vi "Epoxy_Main.vi"() -> ()   [LabVIEW 2020]
doc: "This template is for the Queued Message Handler design pattern.\n\nThe Event Handling Loop generates messages based on user interface actions.\n\nThe Message Handling Loop processes messages generated by the Event Handling Loop, or by other messages. The messages are string values, so new messages can be added easily to the Message Cases case structure in the Message Handling Loop. Each message cluster can also provide an optional value for Message Data, which is a variant that can be converted to whatever message-specific data is required."
uses:
  controls/UI Data.ctl
  DAQLoop_Typedef.ctl
  controls/Data Loop Enum.ctl
  controls/DAQ FGV.ctl
  <vilib>/Utility/error.llb/DialogType.ctl
  controls/Valve Timer FGV.ctl
  controls/SaveTimer.ctl
  Global Loop Stop.vi
  Global Zero or Not Ctrl.vi
  Global Zero Constants.vi
  support/Message Queue/Enqueue Message (Single).vi
  <vilib>/Utility/error.llb/Error Cluster From Error Code.vi
  <vilib>/ErrorRing/Error Ring.xnode
  support/Message Queue/Message Queue.lvlib
  support/User Event - Stop/User Event - Stop.lvlib
  <instrlib>/Agilent 34970/Agilent 34970.lvlib
panel:
  out "T 7":dbl format="%.2f"
  out "T 6":dbl format="%.2f"
  out "T 5":dbl format="%.2f"
  out "T 4":dbl format="%.2f"
  out "T 3":dbl format="%.2f"
  out "T 2":dbl format="%.2f"
  out "T 1":dbl format="%.2f"
  out "Time":string
  out "DAQ":bool
  out "State Execution (ms)":u32=250 format="%.0p"
  out "Messages":string
  out "Lap":dbl format="%<%H:%M:%S>t"
  in  "Interval":dbl=5.0 min=0.0 max=5.0 step=1.0 format="%.2f s"
  in  "FileName":string="Epoxy_"
  in  "Save Command":bool
  in  "Tab Control":enum32{"GRAPH", "OTHER"}(tab)
  in  "Run Interval":dbl=1.0 format="%.1f min"
  in  "Run Auto":bool
  in  "Run B":bool
  in  "Run A":bool
  in  "Axis Update":bool
  out "Waveform Chart Out":dynamicdata(graph)
  in  "Minutes X-axis":dbl format="%#_g min"
  out "Count Down":dbl format="%<%H:%M:%S>t"
  in  "milliseconds DAQ Loop":u32=1000
  in  "Scan List":string="101,102,103,104,105,106,107"
  in  "Transducer Type":T1(ring)
  in  "Thermocouple Type":T2(ring)=enum."T"
  in  "VISA resource name":refnum<visa-resource-name>="COM6"
  out "M1":dbl[](array[numeric])
  in  "Serial Port Configuration":T3={"Timeout Value (10000)"=10000, "Baud Rate (57600)"=enum."9600", "Flow Control (1:XON/XOFF)"=enum."XON / XOFF"}
  in  "Reset (T: Reset)":bool=TRUE
  in  "Save File Headers":string[](array[string])=["T1", "T2", "T3", "T4", "T5", "T6", "T7"]
  in  "Exit":bool
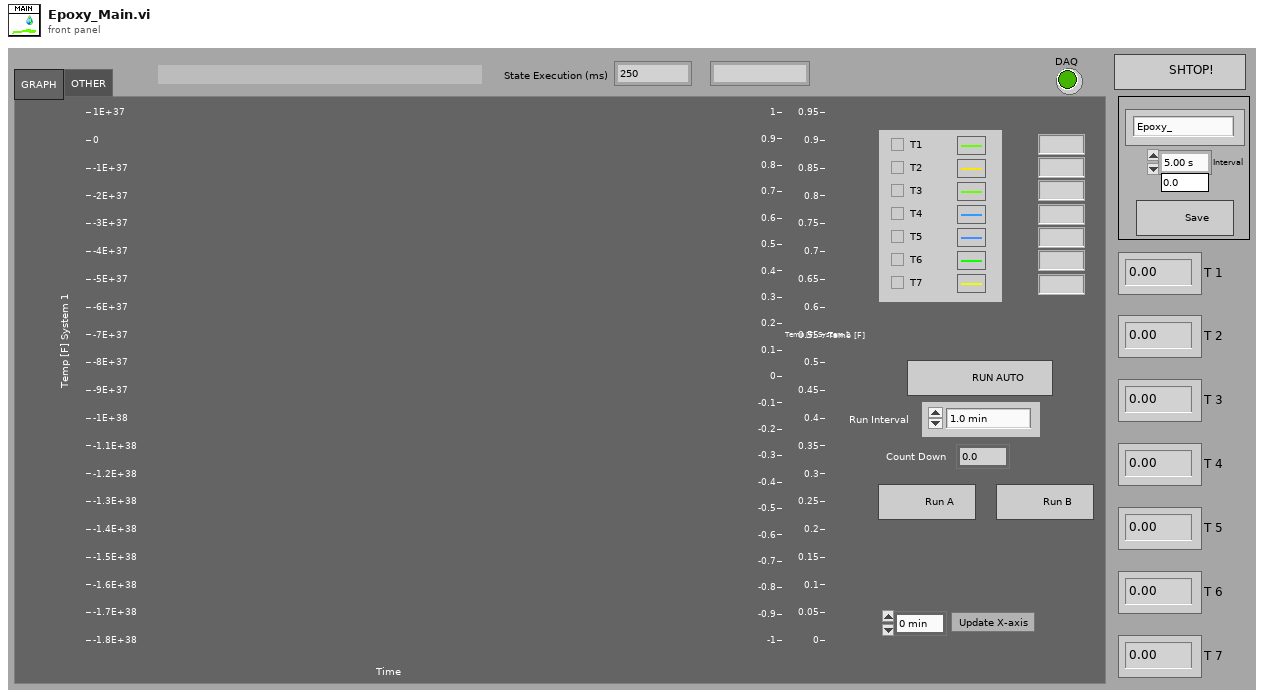
[diagram p1: front panel]
types:
  T1 = enum16{"Thermocouple", "Thermistor", "RTD", "4-Wire RTD", "Default (Last)"}
  T2 = enum16{"B", "E", "J", "K", "N", "R", "S", "T", "Default (Last)"}
  T3 = cluster{"Timeout Value (10000)":u32, "Baud Rate (57600)":enum16{"1200", "2400", "4800", "9600", "19200", "38400", "57600", "115200"}, "Flow Control (1:XON/XOFF)":enum16{"None", "XON / XOFF", "RTS / CTS", "DTR / DSR"}}
  T4 = typedef "Data Loop Enum.ctl" = enum16{"Initialize", "Run", "Exit"}
  T5 = typedef "DAQLoop_Typedef.ctl" = cluster{"XL time":dbl, "Temps":cluster{"TC_1":dbl, "TC_ 2":dbl, "TC_ 3":dbl, "TC_ 4":dbl, "TC_ 5":dbl, "TC_ 6":dbl, "TC_ 7":dbl}}
  T6 = typedef "UI Data.ctl" = cluster{"VISA ref":refnum<visa-resource-name>, "SavePath":path, "tdms file out":refnum<k34>}
  T7 = typedef "Message Queue.lvlib/All Message Queues.ctl" = cluster{"UI":refnum<queue>}
  T8 = typedef "DAQ FGV.ctl" = enum16{"Read", "Pass"}
  T9 = typedef "DialogType.ctl" = u16
  T10 = typedef "Valve Timer FGV.ctl" = enum16{"Run", "Check", "Stop"}
  T11 = typedef "SaveTimer.ctl" = enum16{"Start Save", "StartInterval", "UpdateInterval", "Check"}
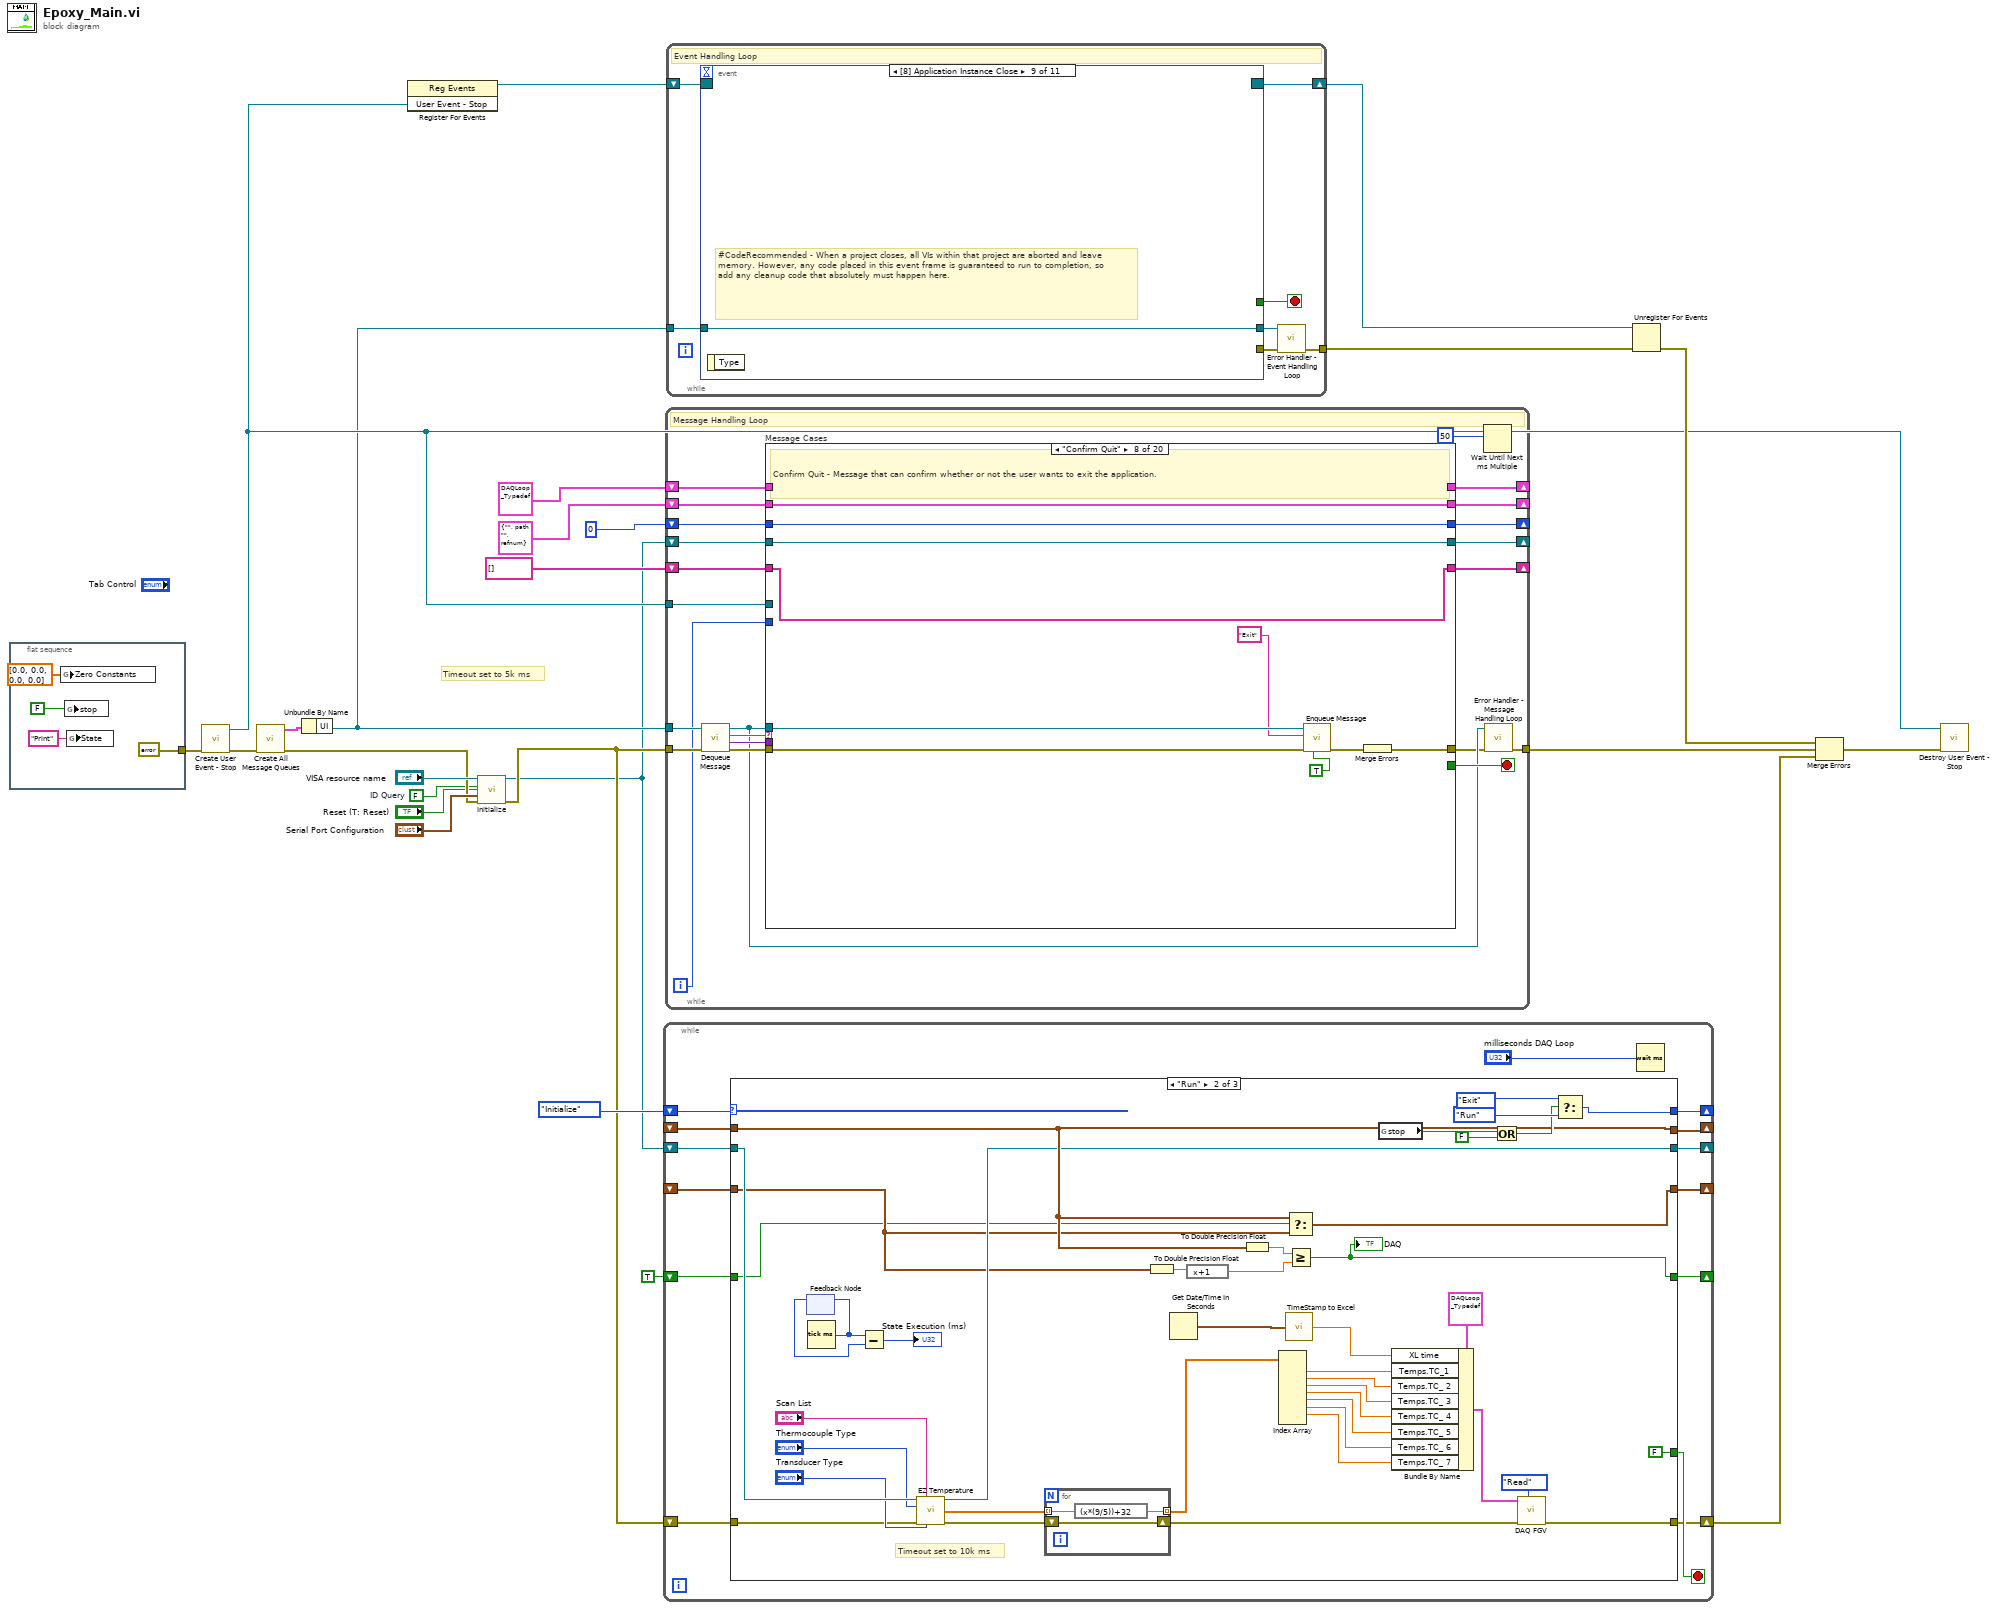
[diagram p0: block diagram]
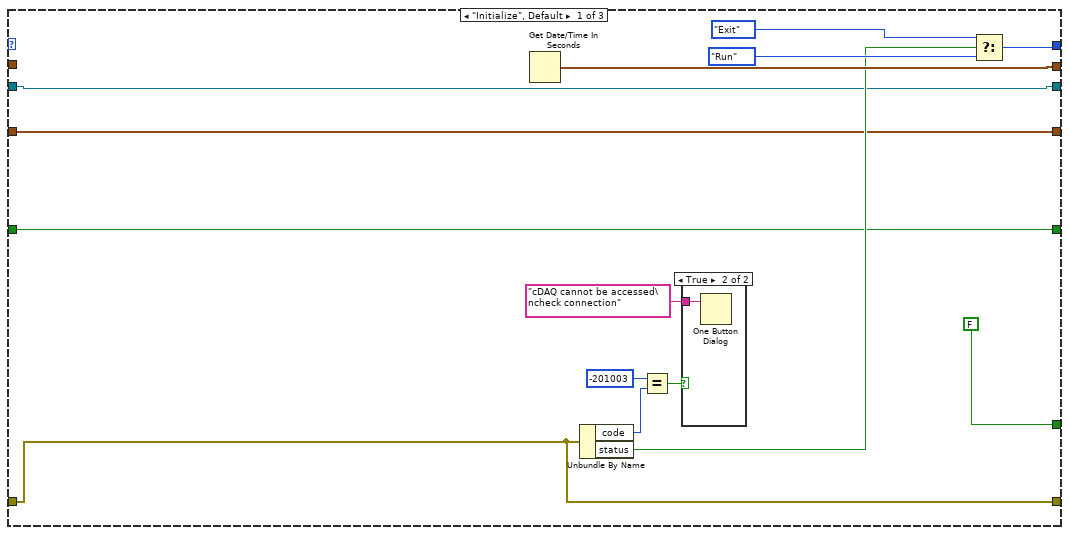
[diagram p2: hidden frame]
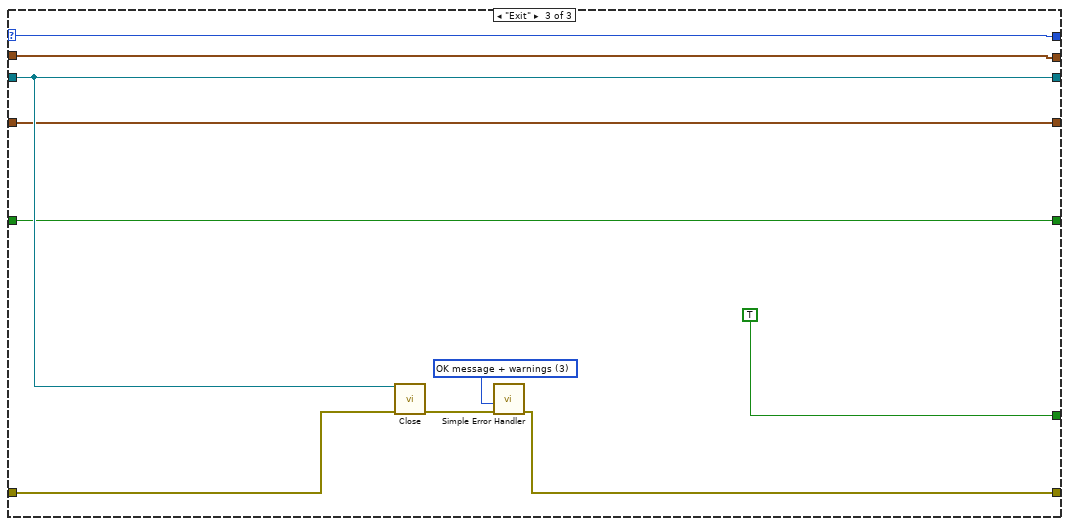
[diagram p4: hidden frame]
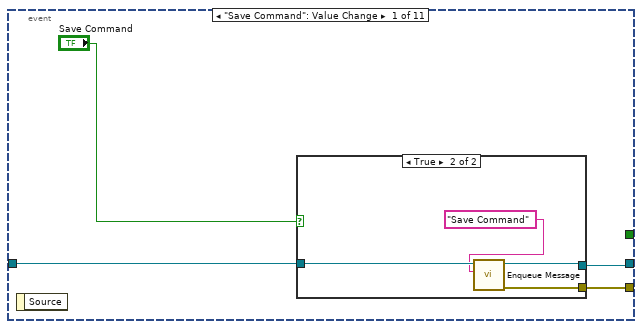
[diagram p5: hidden frame]
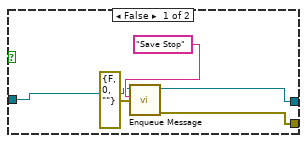
[diagram p6: hidden frame]
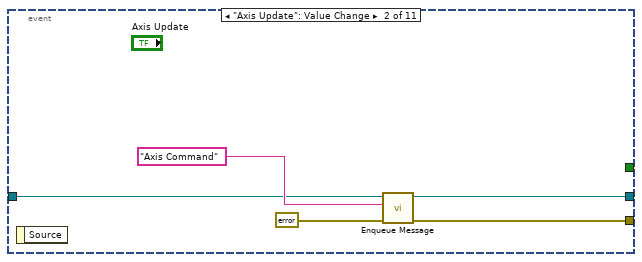
[diagram p7: hidden frame]
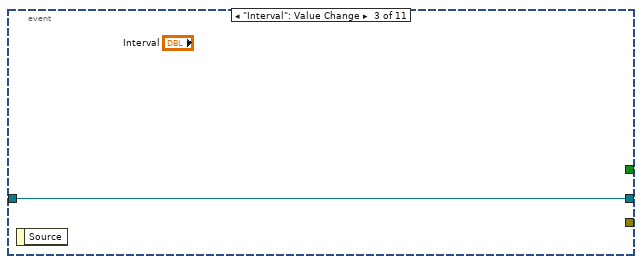
[diagram p8: hidden frame]
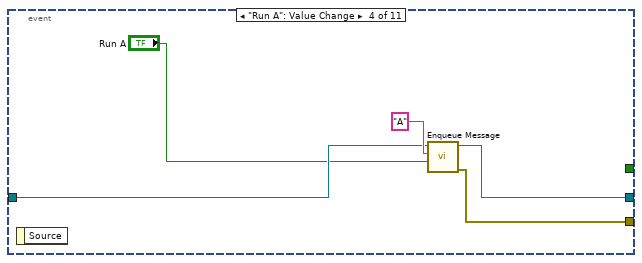
[diagram p9: hidden frame]
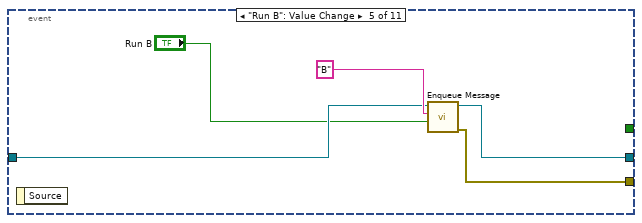
[diagram p10: hidden frame]
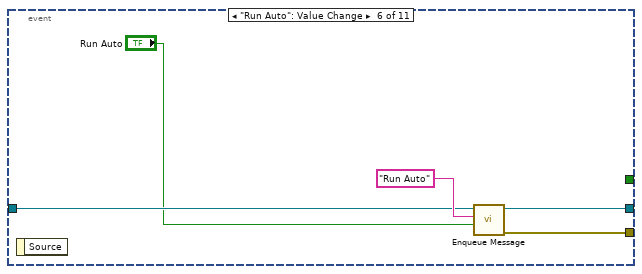
[diagram p11: hidden frame]
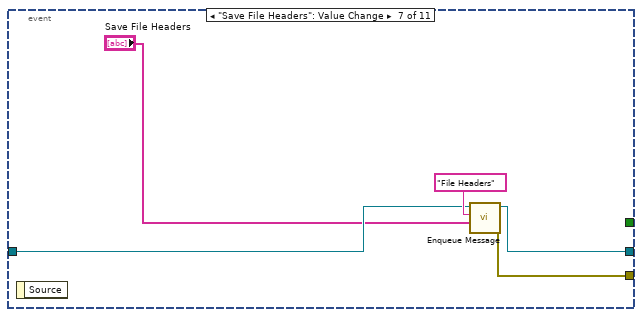
[diagram p12: hidden frame]
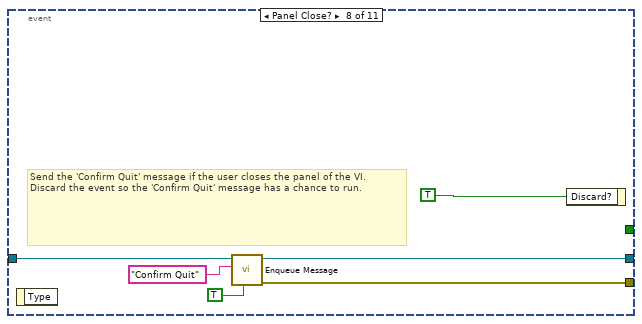
[diagram p13: hidden frame]
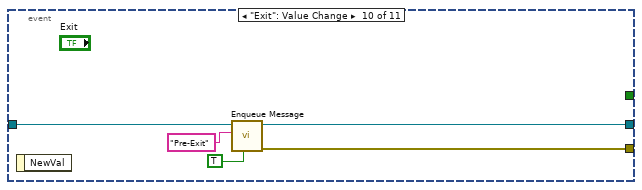
[diagram p14: hidden frame]
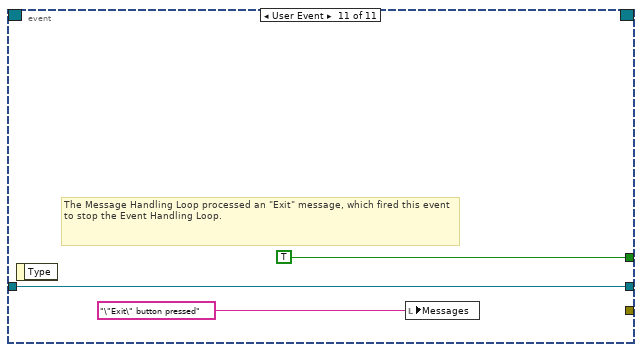
[diagram p15: hidden frame]
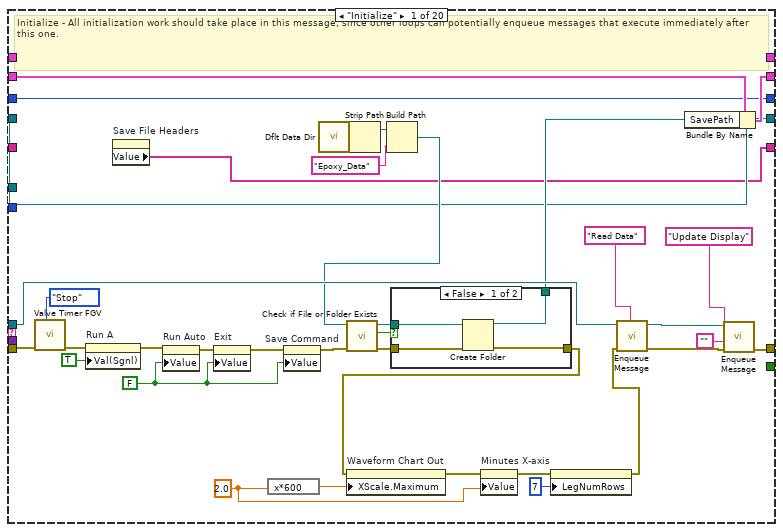
[diagram p16: hidden frame]
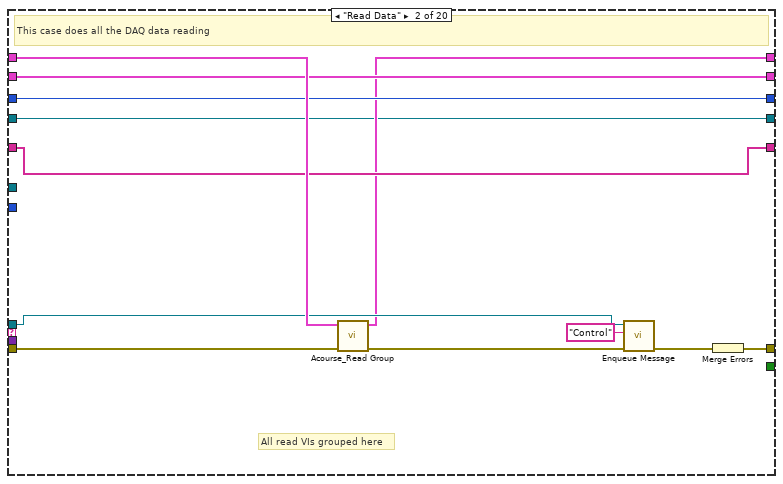
[diagram p18: hidden frame]
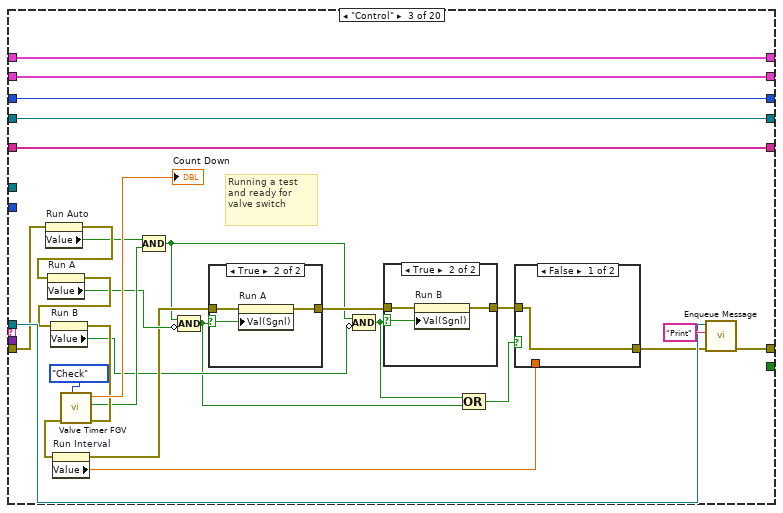
[diagram p19: hidden frame]
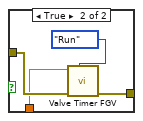
[diagram p20: hidden frame]
diagram:
  w2 = FALSE  # ID Query
  # "Timeout set to 5k ms"
  n1 = flat-sequence {
    tunnel: [errorcluster {"status"=FALSE, "code"=0, "source"=""} ("error out")] -> w16
    frame #0 {
      n2 = global write "Global Zero Constants.vi" "Zero Constants"(dbl[] [0.0, 0.0, 0.0, 0.0] ("Zero Constants")) -> ()
      n3 = global write "Global Loop Stop.vi" "stop"(FALSE ("stop")) -> ()
      n4 = global write "Global Zero or Not Ctrl.vi" "State"("Print" ("State")) -> ()
    }
  }
  n5 = call "Create User Event - Stop.vi"("error in (no error)"=w16) -> ("error out"=w23:errorcluster, "User Event - Stop"=w17:refnum<user-event>)  [unwired: 9 in]
  n6 = call "Create All Message Queues.vi"("error in (no error)"=w23) -> ("error out"=w7:errorcluster, "Message Queues out"=w25:T7)  [unwired: 9 in]
  n7 = Unbundle By Name(w25) -> ("UI"=w15:refnum<queue>)
  n8 = register-events(w17) -> (reference out=w18:refnum<event-registration>)  [unwired: 2 in, 1 out]
  n9 = call <instrlib>:"Initialize.vi"("VISA Resource Name"="VISA resource name", "ID Query (T: Check)"=w2, "Reset (T: Reset)"="Reset (T: Reset)", "Serial Port Configuration"="Serial Port Configuration", "error in (no error)"=w7) -> ("VISA Resource Name Out"=w5:refnum<visa-resource-name>, "error out"=w6:errorcluster)  [unwired: 9 in]
  n10 = while {
    shift-right: [w42] -> _
    shift-left: Data_Loop_Enum."Initialize" ("Enum") -> [w43]
    shift-right: [w34] -> _
    shift-left: w5 -> [w37]
    shift-right: [w36] -> w13
    shift-left: w6 -> [w35]
    shift-right: [w41] -> _
    shift-left: _ -> [w40]
    shift-right: [w32] -> _
    shift-left: _ -> [w33]
    shift-right: [w30] -> _
    shift-left: TRUE -> [w31]
    stop <- w39 stop-if-true
    n11 = case shown="\"Run\"" w43 {
      selector: w43 -> [_ _ w112]
      tunnel: [w47 w91 w107] -> w36
      tunnel: [w46 w77 w106] -> w34
      tunnel: [w55 w92 w112] -> w42
      tunnel: [w54 w84 w111] -> w41
      tunnel: w40 -> [_ w84 w111]
      tunnel: [FALSE FALSE TRUE] -> w39
      tunnel: w37 -> [w46 w80 w106]
      tunnel: w35 -> [w47 w67 w105]
      tunnel: w33 -> [w44 w62 w103]
      tunnel: [w44 w61 w103] -> w32
      tunnel: w31 -> [w45 w60 w104]
      tunnel: [w45 w59 w104] -> w30
      frame "Initialize", Default {
        n12 = Get Date/Time In Seconds() -> (seconds since 1Jan1904=w54:timestamp)
        n13 = Unbundle By Name(w47) -> ("code"=w49:i32, "status"=w48:bool)
        n14 = Equal?(x=-201003, y=w49) -> (x = y?=w51:bool)
        n15 = case shown="True" w51 {
          tunnel: "cDAQ cannot be accessed\ncheck connection" ("message") -> [_ w58]
          frame False {
          }
          frame True {
            n16 = One Button Dialog(message=w58) -> ()  [unwired: 1 in, 1 out]
          }
        }
        n17 = Select(t=Data_Loop_Enum."Exit", s=w48, f=Data_Loop_Enum."Run") -> (s? t:f=w55:T4)
      }
      frame "Run" {
        # "Timeout set to 10k ms"
        n18 = feedback #1() -> (w96:u32)  [unwired: 1 in]
        n19 = Tick Count (ms)() -> (millisecond timer value=w95:u32)
        n20 = feedback-in #1(w95) -> ()
        n21 = Subtract(x=w95, y=w96) -> (x-y=→"State Execution (ms)":u32)
        n22 = call <instrlib>:"EZ Temperature.vi"("VISA Resource Name"=w80, "Scan List (empty)"="Scan List", "Thermocouple Type (8:Def-Last)"="Thermocouple Type", "error in (no error)"=w67, "Transducer Type (4:Def-Last)"="Transducer Type") -> ("VISA Resource Name Out"=w77:refnum<visa-resource-name>, "Output Array"=w64:dbl[], "error out"=w66:errorcluster)  [unwired: 8 in]
        n23 = for {
          shift-right: [w102] -> w65
          shift-left: w66 -> [w102]
          tunnel: w64 -> [w101] mode=indexing
          tunnel: [w100] -> w63 mode=indexing
          n24 = expression code="(x*(9/5))+32"(w101) -> (w100:dbl)
        }
        n25 = To Double Precision Float(number=w62) -> (double precision float=w99:dbl)
        n26 = Get Date/Time In Seconds() -> (seconds since 1Jan1904=w83:timestamp)
        n27 = expression code="x+1"(w99) -> (w97:dbl)
        n28 = To Double Precision Float(number=w84) -> (double precision float=w98:dbl)
        n29 = Index Array(array=w63) -> (element #1=w75:dbl, element #2=w74:dbl, element #3=w73:dbl, element #4=w72:dbl, element #5=w71:dbl, element #6=w70:dbl, element #7=w69:dbl)  [unwired: 8 in, 1 out]
        n30 = call "TimeStamp to Excel.vi"("Time Stamp"=w83) -> ("XL Time"=w68:dbl)
        n31 = Select(t=w84, s=w60, f=w62) -> (s? t:f=w61:timestamp)
        n32 = Greater Or Equal?(x=w98, y=w97) -> (x >= y?=w59:bool)
        "DAQ" <- w59
        n33 = global read "Global Loop Stop.vi" "stop"() -> (w87:bool)
        n34 = Bundle By Name(cluster=T5 {"XL time"=0.0, "Temps"={"TC_1"=0.0, "TC_ 2"=0.0, "TC_ 3"=0.0, "TC_ 4"=0.0, "TC_ 5"=0.0, "TC_ 6"=0.0, "TC_ 7"=0.0}} ("Cluster"), "XL time"=w68, "Temps.TC_1"=w75, "Temps.TC_ 2"=w74, "Temps.TC_ 3"=w73, "Temps.TC_ 4"=w72, "Temps.TC_ 5"=w71, "Temps.TC_ 6"=w70, "Temps.TC_ 7"=w69) -> (w85:T5)
        n35 = Or(x=w87, y=FALSE) -> (x .or. y?=w89:bool)
        n36 = call "DAQ FGV.vi"("Enum"=DAQ_FGV."Read", "error in (no error)"=w65, "Cluster"=w85) -> ("error out"=w91:errorcluster)  [unwired: 7 in, 1 out]
        n37 = Select(t=Data_Loop_Enum."Exit", s=w89, f=Data_Loop_Enum."Run") -> (s? t:f=w92:T4)
      }
      frame "Exit" {
        w109 = T9 3 items=["no dialog", "OK message", "continue or stop message", "OK message + warnings", "continue/stop + warnings"] ("type of dialog (OK msg:1)")
        n38 = call <instrlib>:"Close.vi"("VISA Resource Name"=w106, "error in (no error)"=w105) -> ("error out"=w108:errorcluster)  [unwired: 13 in]
        n39 = call <vilib>:"Simple Error Handler.vi"("type of dialog (OK msg:1)"=w109, "error in (no error)"=w108) -> ("error out"=w107:errorcluster)  [unwired: 3 in, 4 out]
      }
    }
    n40 = Wait (ms)(milliseconds to wait="milliseconds DAQ Loop") -> ()  [unwired: 1 out]
  }
  n41 = while {
    tunnel: w15 -> [w126]
    shift-right: [w133] -> _
    shift-left: T6 {"VISA ref"="", "SavePath"=path "", "tdms file out"=refnum} ("Data Cluster") -> [w134]
    tunnel: w17 -> [w131]
    tunnel: w6 -> [w130]
    tunnel: [w124] -> w24
    shift-right: [w121] -> _
    shift-left: T5 {"XL time"=0.0, "Temps"={"TC_1"=0.0, "TC_ 2"=0.0, "TC_ 3"=0.0, "TC_ 4"=0.0, "TC_ 5"=0.0, "TC_ 6"=0.0, "TC_ 7"=0.0}} ("Cluster") -> [w122]
    shift-right: [w117] -> _
    shift-left: 0 -> [w118]
    shift-right: [w115] -> _
    shift-left: string[] [] ("appended array") -> [w116]
    shift-right: [w113] -> _
    shift-left: w5 -> [w114]
    i -> [w119]
    stop <- w132 stop-if-true
    # "Message Handling Loop"
    n42 = call "Dequeue Message.vi"("error in (no error)"=w130, "Message Queue"=w126) -> ("error out"=w129:errorcluster, "Message Data"=w127:variant, "Message"=w128:string, "dup Message Queue"=w125:refnum<queue>)  [unwired: 6 in]
    n43 = case "Message Cases" shown="\"Confirm Quit\"" w128 {
      selector: w128 -> [_ _ _ _ _ _ _ _ _ _ _ _ _ _ _ _ _ _ _ w489]
      tunnel: w125 -> [w169 w184 w208 w257 w279 _ _ w319 _ _ _ _ _ _ w412 w421 _ w451 w484 _]
      tunnel: w129 -> [w137 w188 w207 w253 w274 w299 w312 w323 w330 w339 w356 w372 w383 w393 w411 w422 w440 w449 w479 _]
      tunnel: [w165 w189 w211 w258 w280 w300 w306 w321 w328 w343 w360 w376 w386 w397 w413 w423 w434 w452 w482 w490] -> w123
      tunnel: w134 -> [w163 w183 w217 w259 w289 w301 w311 w322 w329 w344 w361 w377 w387 w398 w403 w430 w439 w450 w473 w491]
      tunnel: [w162 w183 w217 w259 w289 w301 w311 w322 w329 w344 w361 w377 w387 w398 w402 w430 w439 w450 w473 w491] -> w133
      tunnel: [_ _ _ _ _ _ _ _ _ _ _ _ _ _ _ _ _ _ TRUE _] -> w132
      tunnel: w127 -> [_ _ _ _ _ w298 w310 _ _ _ w355 w371 w382 _ _ _ _ _ w476 _]
      tunnel: w131 -> [_ _ _ _ _ _ _ _ _ _ _ _ _ _ _ _ _ _ w481 _]
      tunnel: w122 -> [w171 w187 w216 w250 w290 w295 w305 w316 w327 w342 w359 w375 w385 w396 w417 w429 w441 w454 w474 w488]
      tunnel: [w171 w180 w216 w250 w290 w295 w305 w316 w327 w342 w359 w375 w385 w396 w417 w429 w441 w454 w474 w488] -> w121
      tunnel: w119 -> [_ _ _ _ _ _ _ _ _ _ _ _ _ _ _ w427 _ _ _ _]
      tunnel: w118 -> [w143 w182 w215 w255 w277 w293 w304 w315 w326 w341 w358 w374 w384 w395 w401 _ w433 w448 w472 w487]
      tunnel: [w143 w182 w215 w255 w277 w293 w304 w315 w326 w341 w358 w374 w384 w395 w401 w425 w433 w448 w472 w487] -> w117
      tunnel: w116 -> [_ w181 w214 w237 w276 w292 w303 w314 w325 w340 w357 w373 _ w390 w400 w419 w432 w447 w471 w486]
      tunnel: [w135 w181 w214 w237 w276 w292 w303 w314 w325 w340 w357 w373 w378 w390 w400 w419 w432 w447 w471 w486] -> w115
      tunnel: w114 -> [w144 w179 w213 w231 w275 w291 w302 w313 w324 w333 w348 w369 w381 w389 w399 w418 w431 w446 w469 w485]
      tunnel: [w144 w179 w213 w231 w275 w291 w302 w313 w324 w334 w347 w369 w381 w389 w399 w418 w431 w446 w469 w485] -> w113
      frame "Initialize" {
        w148 = 2.0 ("X Scale.Range:Maximum")
        w139 = FALSE ("Exit")
        # "Initialize - All initialization work should take place in this message, since other loops can potentially enqueue messages that execute immediately after this one."
        n44 = call "Valve Timer FGV.vi"("Valve Timer Enum"=Valve_Timer_FGV."Stop", "error in (no error)"=w137) -> ("error out"=w138:errorcluster)  [unwired: 7 in, 2 out]
        n45 = property on="Run A" class="Bool (strict)"(error in=w138, "Val(Sgnl)"=TRUE ("Value (Signaling)")) -> (error out=w141:errorcluster)  [unwired: 1 in, 1 out]
        n46 = property on="Save File Headers" class="Arr (strict)"() -> ("Value"=w135:string[])  [unwired: 2 in, 2 out]
        n47 = property on="Run Auto" class="Bool (strict)"(error in=w141, "Value"=w139) -> (error out=w140:errorcluster)  [unwired: 1 in, 1 out]
        n48 = property on="Exit" class="Bool (strict)"(error in=w140, "Value"=w139) -> (error out=w153:errorcluster)  [unwired: 1 in, 1 out]
        n49 = expression code="x*600"(w148) -> (w150:dbl)
        n50 = property on="Save Command" class="Bool (strict)"(error in=w153, "Value"=w139) -> (error out=w152:errorcluster)  [unwired: 1 in, 1 out]
        n51 = call <vilib>:"Dflt Data Dir.vi"() -> ("App:Default Data Directory"=w161:path)
        n52 = Strip Path(path=w161) -> (stripped path=w160:path)  [unwired: 1 out]
        n53 = Build Path(base path=w160, name or relative path="Epoxy_Data") -> (appended path=w158:path)
        n54 = call <vilib>:"Check if File or Folder Exists.vi"("error in (no error)"=w152, "path"=w158) -> ("error out"=w157:errorcluster, "file or folder exists?"=w156:bool, "dup path"=w155:path)  [unwired: 7 in]
        n55 = case shown="False" w156 {
          tunnel: w157 -> [w174 w176]
          tunnel: w155 -> [w175 w177]
          tunnel: [w172 w177] -> w154
          tunnel: [w173 w176] -> w151
          frame False {
            n56 = Create Folder(path (use dialog)=w175, error in=w174) -> (created path=w172:path, error out=w173:errorcluster)  [unwired: 1 in, 1 out]
          }
          frame True {
          }
        }
        n57 = property on="Waveform Chart Out" class="WFChart (strict)"(error in=w151, "XScale.Maximum"=w150) -> (error out=w149:errorcluster)  [unwired: 1 in, 1 out]
        n58 = property on="Minutes X-axis" class="DigNum (strict)"(error in=w149, "Value"=w148) -> (error out=w147:errorcluster)  [unwired: 1 in, 1 out]
        n59 = property on="Waveform Chart Out" class="WFChart (strict)"(error in=w147, "LegNumRows"=u32 7 ("Legend:Number of Rows")) -> (error out=w146:errorcluster)  [unwired: 1 in, 1 out]
        n60 = call-poly "Enqueue Message.vi"("error in (no error)"=w146, "Message"="Read Data", "Message Queue"=w169) -> ("error out"=w166:errorcluster, "dup Message Queue"=w167:refnum<queue>)  [unwired: 7 in]
        n61 = Bundle By Name(cluster=w163, "SavePath"=w154) -> (w162:T6)
        n62 = call-poly "Enqueue Message.vi"("error in (no error)"=w166, "Message Data"="", "Message"="Update Display", "Message Queue"=w167) -> ("error out"=w165:errorcluster)  [unwired: 6 in, 1 out]
      }
      frame "Read Data" {
        # "All read VIs grouped here"
        # "This case does all the DAQ data reading"
        n63 = call "Acourse_Read Group.vi"("error in (no error)"=w188, "Cluster in"=w187) -> ("error out"=w186:errorcluster, "Cluster out"=w180:T5)  [unwired: 8 in]
        n64 = call-poly "Enqueue Message.vi"("error in (no error)"=w186, "Message"="Control", "Message Queue"=w184) -> ("error out"=w185:errorcluster)  [unwired: 7 in, 1 out]
        n65 = Merge Errors(w185) -> (w189:errorcluster)
      }
      frame "Control" {
        # "Running a test and ready for valve switch"
        n66 = property on="Run Auto" class="Bool (strict)"(error in=w207) -> (error out=w206:errorcluster, "Value"=w202:bool)  [unwired: 1 in, 1 out]
        n67 = property on="Run A" class="Bool (strict)"(error in=w206) -> (error out=w205:errorcluster, "Value"=w200:bool)  [unwired: 1 in, 1 out]
        n68 = property on="Run B" class="Bool (strict)"(error in=w205) -> (error out=w204:errorcluster, "Value"=w194:bool)  [unwired: 1 in, 1 out]
        n69 = call "Valve Timer FGV.vi"("Valve Timer Enum"=Valve_Timer_FGV."Check", "error in (no error)"=w204) -> ("error out"=w203:errorcluster, "Switch Valve"=w201:bool, "Count Down [s]"=→"Count Down":dbl)  [unwired: 7 in]
        n70 = property on="Run Interval" class="DigNum (strict)"(error in=w203) -> (error out=w199:errorcluster, "Value"=w190:dbl)  [unwired: 1 in, 1 out]
        n71 = Compound Arithmetic op=AND(w202, w201) -> (w195:bool)
        n72 = Compound Arithmetic op=AND(w195, invert w200) -> (w193:bool)
        n73 = case shown="True" w193 {
          selector: w193 -> [_ w230]
          tunnel: w199 -> [w227 w229]
          tunnel: [w227 w228] -> w198
          frame False {
          }
          frame True {
            n74 = property on="Run A" class="Bool (strict)"(error in=w229, "Val(Sgnl)"=w230) -> (error out=w228:errorcluster)  [unwired: 1 in, 1 out]
          }
        }
        n75 = Compound Arithmetic op=AND(w195, invert w194) -> (w192:bool)
        n76 = case shown="True" w192 {
          selector: w192 -> [_ w224]
          tunnel: w198 -> [w223 w226]
          tunnel: [w223 w225] -> w197
          frame False {
          }
          frame True {
            n77 = property on="Run B" class="Bool (strict)"(error in=w226, "Val(Sgnl)"=w224) -> (error out=w225:errorcluster)  [unwired: 1 in, 1 out]
          }
        }
        n78 = Compound Arithmetic op=OR(w192, w193) -> (w191:bool)
        n79 = case shown="False" w191 {
          tunnel: w197 -> [w218 w221]
          tunnel: [w218 w220] -> w196
          tunnel: w190 -> [_ w219]
          frame False {
          }
          frame True {
            n80 = call "Valve Timer FGV.vi"("Valve Timer Enum"=Valve_Timer_FGV."Run", "error in (no error)"=w221, "Duration(min)"=w219) -> ("error out"=w220:errorcluster)  [unwired: 6 in, 2 out]
          }
        }
        n81 = call-poly "Enqueue Message.vi"("error in (no error)"=w196, "Message"="Print", "Message Queue"=w208) -> ("error out"=w211:errorcluster)  [unwired: 7 in, 1 out]
      }
      frame "Print" {
        # "If the Save button is pressed, the save\nstate is enqued"
        # "In this state data is displayed on screen"
        n82 = Unbundle By Name(w250) -> ("Temps.TC_1"=w240:dbl, "Temps.TC_ 2"=w239:dbl, "Temps.TC_ 3"=w238:dbl, "Temps.TC_ 4"=w235:dbl, "Temps.TC_ 5"=w234:dbl, "Temps.TC_ 6"=w233:dbl, "Temps.TC_ 7"=w232:dbl)
        "T 1" <- w240
        "T 2" <- w239
        "T 3" <- w238
        "T 4" <- w235
        "T 5" <- w234
        "T 6" <- w233
        "T 7" <- w232
        n83 = Tick Count (ms)() -> (millisecond timer value=w249:u32)
        n84 = feedback-in #2(w249) -> ()
        n85 = feedback #2() -> (w248:u32)  [unwired: 1 in]
        n86 = Build Array(w240, w239, w238, w235, w234, w233, w232) -> (w242:dbl[])
        n87 = Subtract(x=w249, y=w248) -> (x-y=w247:u32)
        n88 = To Double Precision Float(number=w247) -> (double precision float=w246:dbl)
        n89 = call "Convert to Dynamic Data"("Array"=w242) -> ("Dynamic Data Type"=→"Waveform Chart Out":dynamicdata)  [unwired: 3 in]
        n90 = Array Size(array=w242) -> (size(s)=w236:i32)
        n91 = expression code="x/1000"(w246) -> ()  [unwired: 1 out]
        n92 = Array Subset(array=w242, index=w236) -> (→"M1":dbl[])  [unwired: 1 in]
        n93 = for {
          N: w236 -> [_]
          shift-right: [w263] -> w254
          shift-left: w253 -> [w264]
          tunnel: w237 -> [w261] mode=indexing
          tunnel: u32[] [0, 0, 0, 1, 1, 1, 2] -> [w260] mode=indexing
          i -> [w262]
          n94 = property on="Waveform Chart" class="WFChart (strict)"(error in=w264, "Active Plot"=w262, "Plot.YScaleIdx"=w260, "Plot.Plot Name"=w261) -> (error out=w263:errorcluster)  [unwired: 1 in, 1 out]
        }
        n95 = Get Date/Time In Seconds() -> (seconds since 1Jan1904=w245:timestamp)
        n96 = Get Date/Time String(seconds (now)=w245, want seconds? (F)=TRUE) -> (time string=→"Time":string)  [unwired: 1 in, 1 out]
        n97 = call-poly "Enqueue Message.vi"("error in (no error)"=w254, "Message"="Save", "Message Queue"=w257) -> ("error out"=w258:errorcluster)  [unwired: 7 in, 1 out]
      }
      frame "Save" {
        # "Save data to the file created in the \"Save Command Case\""
        n98 = property on="Run A" class="Bool (strict)"(error in=w274) -> (error out=w273:errorcluster, "Value"=w271:bool)  [unwired: 1 in, 1 out]
        n99 = property on="Run B" class="Bool (strict)"(error in=w273) -> (error out=w272:errorcluster, "Value"=w270:bool)  [unwired: 1 in, 1 out]
        n100 = Boolean To (0,1)(Boolean=w271) -> (0, 1=w269:i16)
        n101 = Boolean To (0,1)(Boolean=w270) -> (0, 1=w268:i16)
        n102 = To Double Precision Float(number=w269) -> (double precision float=w267:dbl)
        n103 = To Double Precision Float(number=w268) -> (double precision float=w266:dbl)
        n104 = Build Array(w267, w266) -> (w265:dbl[])
        n105 = call "Epoxy_SaveTimer.vi"("Enum"=SaveTimer."Check", "error in (no error)"=w272) -> ("error out"=w288:errorcluster, "Int Lap [s]"=w284:dbl, "Int Done?"=w286:bool, "Saving?"=w285:bool)  [unwired: 6 in]
        n106 = Select(t=w284, s=w285, f=0.0) -> (s? t:f=→"Lap":dbl)
        n107 = call "Epoxy_Save.vi"("Valve A, B"=w265, "Labels"=w276, "error in (no error)"=w288, "Int Done?"=w286, "Data Cluster"=w289, "Cluster"=w290) -> ("error out"=w278:errorcluster)  [unwired: 5 in]
        n108 = call-poly "Enqueue Message.vi"("error in (no error)"=w278, "Message"="Read Data", "Message Queue"=w279) -> ("error out"=w280:errorcluster)  [unwired: 7 in, 1 out]
      }
      frame "Update Display" {
        # "Update Display - Convert the message data to a string to display in the Data Display indicator."
        n109 = Variant To Data(error in=w299, type="", Variant=w298) -> (data=→"Messages":string, error out=w296:errorcluster)
        n110 = Merge Errors(w296) -> (w300:errorcluster)
      }
      frame "Error" {
        # "Error - Display an error dialog. This message is sent by the \"Error Handler\" VIs at the end of other loops in this application."
        n111 = Variant To Data(error in=w312, type=errorcluster {"status"=FALSE, "code"=0, "source"=""} ("error constant"), Variant=w310) -> (data=w308:errorcluster, error out=w307:errorcluster)
        n112 = call <vilib>:"Simple Error Handler.vi"("error in (no error)"=w308) -> ()  [unwired: 4 in, 5 out]
        n113 = Merge Errors(w307) -> (w306:errorcluster)
      }
      frame "Confirm Quit" {
        # "Confirm Quit - Message that can confirm whether or not the user wants to exit the application."
        n114 = call-poly "Enqueue Message.vi"("Priority Message? (F)"=TRUE, "error in (no error)"=w323, "Message"="Exit", "Message Queue"=w319) -> ("error out"=w320:errorcluster)  [unwired: 6 in, 1 out]
        n115 = Merge Errors(w320) -> (w321:errorcluster)
      }
      frame "---Copy This Frame---" {
        # "Duplicate this frame when creating new messages.  Change this comment in the duplicated frame to describe this message."
        n116 = Merge Errors(w330) -> (w328:errorcluster)
      }
      frame "A" {
        w331 = "213,215"  # B Valves
        w332 = "214,216"  # A Valves
        # "TRUE IS A"
        # "Duplicate this frame when creating new messages.  Change this comment in the duplicated frame to describe this message."
        n117 = property on="Run B" class="Bool (strict)"(error in=w339, "Value"=FALSE ("Run B")) -> (error out=w337:errorcluster)  [unwired: 1 in, 1 out]
        n118 = call "Valve Control VI.vi"("Boolean"=TRUE, "error in (no error)"=w337, "B Valves"=w331, "A Valves"=w332, "VISA Refnum in"=w333) -> ("error out"=w336:errorcluster, "VISA Resource Name Out"=w334:refnum<visa-resource-name>)  [unwired: 5 in]
        n119 = Merge Errors(w336) -> (w343:errorcluster)
      }
      frame "B" {
        w345 = "213,215"  # B Valves
        w346 = "214,216"  # A Valves
        # "TRUE IS A"
        # "Duplicate this frame when creating new messages.  Change this comment in the duplicated frame to describe this message."
        n120 = Variant To Data(error in=w356, type=TRUE, Variant=w355) -> (error out=w353:errorcluster)  [unwired: 1 out]
        n121 = property on="Run A" class="Bool (strict)"(error in=w353, "Value"=FALSE ("Run A")) -> (error out=w350:errorcluster)  [unwired: 1 in, 1 out]
        n122 = call "Valve Control VI.vi"("Boolean"=FALSE, "error in (no error)"=w350, "B Valves"=w345, "A Valves"=w346, "VISA Refnum in"=w348) -> ("error out"=w351:errorcluster, "VISA Resource Name Out"=w347:refnum<visa-resource-name>)  [unwired: 5 in]
        n123 = Merge Errors(w351) -> (w360:errorcluster)
      }
      frame "Run Auto" {
        # "Duplicate this frame when creating new messages.  Change this comment in the duplicated frame to describe this message."
        n124 = Variant To Data(error in=w372, type=TRUE, Variant=w371) -> (data=w366:bool, error out=w368:errorcluster)
        n125 = Select(t=Valve_Timer_FGV."Run" ("Valve Timer Enum"), s=w366, f=Valve_Timer_FGV."Stop") -> (s? t:f=w363:T10)
        n126 = call "Valve Timer FGV.vi"("Valve Timer Enum"=w363, "error in (no error)"=w368, "Duration(min)"="Run Interval") -> ("error out"=w367:errorcluster)  [unwired: 6 in, 2 out]
        n127 = Merge Errors(w367) -> (w376:errorcluster)
      }
      frame "File Headers" {
        # "Duplicate this frame when creating new messages.  Change this comment in the duplicated frame to describe this message."
        n128 = Variant To Data(error in=w383, type=string[] ["T1", "T2", "T3", "T4", "T5", "T6", "T7"] ("Save File Headers"), Variant=w382) -> (data=w378:string[], error out=w380:errorcluster)
        n129 = Merge Errors(w380) -> (w386:errorcluster)
      }
      frame "Axis Command" {
        # "I know weird but\nthis will give you minutes"
        # "Duplicate this frame when creating new messages.  Change this comment in the duplicated frame to describe this message."
        n130 = control-ref of="Waveform Chart Out"() -> (w391:refnum<vi>)
        n131 = expression code="x*600"("Minutes X-axis") -> (w388:dbl)
        n132 = property on="Property Node" class="WFChart (strict)"(reference=w391, error in=w393, "XScale.Maximum"=w388) -> (error out=w392:errorcluster)  [unwired: 1 out]
        n133 = Merge Errors(w392) -> (w397:errorcluster)
      }
      frame "Save Command" {
        # "Setup save location"
        # "Execute Save after this state"
        # "Saving headers for our data file, this case is executed when the Save Button is pressed in the UI"
        n134 = call "Epoxy_SaveTimer.vi"("Enum"=SaveTimer."Start Save", "error in (no error)"=w411, "Save?"=TRUE) -> ("error out"=w404:errorcluster)  [unwired: 5 in, 3 out]
        n135 = property on="Interval" class="DigNum (strict)"(error in=w404) -> (error out=w406:errorcluster, "Value"=w405:dbl)  [unwired: 1 in, 1 out]
        n136 = call "Epoxy_SaveTimer.vi"("Enum"=SaveTimer."StartInterval", "error in (no error)"=w406, "Interval"=w405) -> ("error out"=w407:errorcluster)  [unwired: 5 in, 3 out]
        n137 = call "TDMS Reference Create.vi"("error in (no error)"=w407, "FileName"="FileName", "Refs"=w403) -> ("error out"=w414:errorcluster, "Refs Out"=w402:T6)  [unwired: 7 in]
        n138 = call-poly "Enqueue Message.vi"("error in (no error)"=w414, "Message"="Save", "Message Queue"=w412) -> ("error out"=w413:errorcluster)  [unwired: 7 in, 1 out]
      }
      frame "Zero Command" {
        n139 = Add(x=10000, y=w427) -> (x+y=w425:i32)
        n140 = global write "Global Zero or Not Ctrl.vi" "State"("Zero" ("State")) -> ()
        n141 = call-poly "Enqueue Message.vi"("Priority Message? (F)"=TRUE, "error in (no error)"=w422, "Message"="Read Data", "Message Queue"=w421) -> ("error out"=w423:errorcluster)  [unwired: 6 in, 1 out]
      }
      frame "Save Stop" {
        # "Save the header\nto a CSV file"
        # "Execute Save after this state"
        # "This location should be a folder \"EpoxyData\" created on your \"MyDocuments Folder\", replace SSO with your own"
        # "Saving headers for our data file, this case is executed when the Save Button is pressed in the UI"
        n142 = Unbundle By Name(w439) -> ("tdms file out"=w438:refnum<k34>)
        n143 = TDMS Close(8:w440, 11:w438) -> (0:w435:errorcluster)  [unwired: 1 out]
        n144 = call "Epoxy_SaveTimer.vi"("Enum"=SaveTimer."Start Save", "error in (no error)"=w435, "Save?"=FALSE) -> ("error out"=w434:errorcluster)  [unwired: 5 in, 3 out]
      }
      frame "Pre-Exit" {
        w444 = FALSE ("Start Cycle")
        # "Turn everything off before exiting"
        n145 = property on="Save Command" class="Bool (strict)"(error in=w449, "Value"=w444) -> (error out=w445:errorcluster)  [unwired: 1 in, 1 out]
        n146 = Not(x=w444) -> (.not. x?=w442:bool)
        n147 = disable-structure shown="Disabled" {
          disable-tunnel: w446 -> [w458 _]
          disable-tunnel: w445 -> [w457 w468]
          disable-tunnel: [w456 w468] -> w443
          disable-tunnel: w442 -> [w455 _]
          frame Disabled {
            n148 = call <instrlib>:"Switch.vi"("Channel List(empty)"="215", "error in (no error)"=w457, "Open/Close (F:Close)"=w455, "VISA Resource Name"=w458) -> ("error out"=w464:errorcluster)  [unwired: 5 in, 2 out]
            n149 = call <instrlib>:"Switch.vi"("Channel List(empty)"="213", "error in (no error)"=w464, "VISA Resource Name"=w458) -> ("error out"=w461:errorcluster, "VISA Resource Name Out"=w462:refnum<visa-resource-name>)  [unwired: 6 in, 1 out]
            n150 = call <instrlib>:"Switch.vi"("Channel List(empty)"="216", "error in (no error)"=w461, "Open/Close (F:Close)"=w455, "VISA Resource Name"=w462) -> ("error out"=w460:errorcluster, "VISA Resource Name Out"=w459:refnum<visa-resource-name>)  [unwired: 5 in, 1 out]
            n151 = call <instrlib>:"Switch.vi"("Channel List(empty)"="214", "error in (no error)"=w460, "Open/Close (F:Close)"=w455, "VISA Resource Name"=w459) -> ("error out"=w456:errorcluster)  [unwired: 5 in, 2 out]
          }
          frame Enabled {
          }
        }
        n152 = call-poly "Enqueue Message.vi"("error in (no error)"=w443, "Message"="Exit", "Message Queue"=w451) -> ("error out"=w452:errorcluster)  [unwired: 7 in, 1 out]
      }
      frame "Exit" {
        # "Stop the VI"
        # "Release the message queue reference"
        # "Exit - Exit the application."
        n153 = Release Queue(queue=w484, error in (no error)=w479) -> (error out=w470:errorcluster)  [unwired: 1 in, 2 out]
        n154 = Variant To Data(type=errorcluster {"status"=FALSE, "code"=0, "source"=""} ("error constant"), Variant=w476) -> (data=w477:errorcluster)  [unwired: 1 in, 1 out]
        n155 = call <vilib>:"Simple Error Handler.vi"("error in (no error)"=w477) -> ()  [unwired: 4 in, 5 out]
        n156 = call "Fire User Event - Stop.vi"("User Event - Stop"=w481) -> ("error out"=w480:errorcluster)  [unwired: 10 in]
        n157 = global write "Global Loop Stop.vi" "stop"(TRUE ("stop")) -> ()
        n158 = Merge Errors(w480, w470) -> (w482:errorcluster)
      }
      frame Default {
        # "'Default' case only runs if there is a message that isn't defined in any of the other cases.  Output a programming error."
        n159 = xnode "Error Ring"("parameter 0"=w489) -> ("error out"=w490:errorcluster)
      }
    }
    n160 = Wait Until Next ms Multiple(millisecond multiple=u32 50) -> ()  [unwired: 1 out]
    n161 = call "Error Handler - Message Handling Loop.vi"("error in (no error)"=w123, "Message Queue"=w125) -> ("dup error in"=w124:errorcluster)  [unwired: 8 in, 1 out]
  }
  n162 = while {
    tunnel: w15 -> [w505]
    shift-right: [w503] -> w20
    shift-left: w18 -> [w504]
    tunnel: [w499] -> w4
    stop <- w501 stop-if-true
    # "Event Handling Loop"
    n163 = event shown="[8] Application Instance Close" {
      selector: w504 -> [_ _ _ _ _ _ _ _ _ _ _]
      dyn-events: [_ _ _ _ _ _ _ _ _ _ _] -> w503
      timeout: _ -> [_ _ _ _ _ _ _ _ _ _ _]
      tunnel: [_ _ _ _ _ _ _ _ _ _ TRUE ("Discard?")] -> w501
      tunnel: w505 -> [w509 w522 w524 w528 w533 w537 w543 w549 w551 w556 w559]
      tunnel: [w508 w519 _ w526 w531 w535 w541 w548 _ w555 _] -> w502
      tunnel: [w507 w521 w524 w527 w532 w538 w542 w547 w551 w554 w559] -> w500
      event "Save Command": Value Change {
        n164 = event-data() -> ()  [unwired: 1 in, 1 out]
        n165 = case shown="True" "Save Command" {
          tunnel: w509 -> [w511 w518]
          tunnel: [w512 w517] -> w508
          tunnel: [w513 w515] -> w507
          frame False {
            n166 = call-poly "Enqueue Message.vi"("error in (no error)"=errorcluster {"status"=FALSE, "code"=0, "source"=""}, "Message"="Save Stop", "Message Queue"=w511) -> ("error out"=w512:errorcluster, "dup Message Queue"=w513:refnum<queue>)  [unwired: 7 in]
          }
          frame True {
            n167 = call-poly "Enqueue Message.vi"("Message"="Save Command", "Message Queue"=w518) -> ("error out"=w517:errorcluster, "dup Message Queue"=w515:refnum<queue>)  [unwired: 8 in]
          }
        }
      }
      event "Axis Update": Value Change {
        n168 = event-data() -> ()  [unwired: 1 in, 1 out]
        n169 = call-poly "Enqueue Message.vi"("error in (no error)"=errorcluster {"status"=FALSE, "code"=0, "source"=""}, "Message"="Axis Command", "Message Queue"=w522) -> ("error out"=w519:errorcluster, "dup Message Queue"=w521:refnum<queue>)  [unwired: 7 in]
      }
      event "Interval": Value Change {
        n170 = event-data() -> ()  [unwired: 1 in, 1 out]
      }
      event "Run A": Value Change {
        n171 = event-data() -> ()  [unwired: 1 in, 1 out]
        n172 = call-poly "Enqueue Message.vi"("Message Data"="Run A", "Message"="A", "Message Queue"=w528) -> ("error out"=w526:errorcluster, "dup Message Queue"=w527:refnum<queue>)  [unwired: 7 in]
      }
      event "Run B": Value Change {
        n173 = event-data() -> ()  [unwired: 1 in, 1 out]
        n174 = call-poly "Enqueue Message.vi"("Message Data"="Run B", "Message"="B", "Message Queue"=w533) -> ("error out"=w531:errorcluster, "dup Message Queue"=w532:refnum<queue>)  [unwired: 7 in]
      }
      event "Run Auto": Value Change {
        n175 = event-data() -> ()  [unwired: 1 in, 1 out]
        n176 = call-poly "Enqueue Message.vi"("Message Data"="Run Auto", "Message"="Run Auto", "Message Queue"=w537) -> ("error out"=w535:errorcluster, "dup Message Queue"=w538:refnum<queue>)  [unwired: 7 in]
      }
      event "Save File Headers": Value Change {
        n177 = event-data() -> ()  [unwired: 1 in, 1 out]
        n178 = call-poly "Enqueue Message.vi"("Message Data"="Save File Headers", "Message"="File Headers", "Message Queue"=w543) -> ("error out"=w541:errorcluster, "dup Message Queue"=w542:refnum<queue>)  [unwired: 7 in]
      }
      event Panel Close? {
        # "Send the 'Confirm Quit' message if the user closes the panel of the VI. Discard the event so the 'Confirm Quit' message has a chance to run."
        n179 = event-data() -> ()  [unwired: 1 in, 1 out]
        n180 = call-poly "Enqueue Message.vi"("Priority Message? (F)"=TRUE, "Message"="Confirm Quit", "Message Queue"=w549) -> ("error out"=w548:errorcluster, "dup Message Queue"=w547:refnum<queue>)  [unwired: 7 in]
        n181 = event-data("Discard?"=TRUE) -> ()  [unwired: 1 in, 1 out]
      }
      event Application Instance Close {
        # "#CodeRecommended - When a project closes, all VIs within that project are aborted and leave memory. However, any code placed in this event frame is guaranteed to run to completion, so add any cleanup code that absolutely must happen here."
        n182 = event-data() -> ()  [unwired: 1 in, 1 out]
      }
      event "Exit": Value Change {
        n183 = event-data() -> ()  [unwired: 1 in, 1 out]
        n184 = call-poly "Enqueue Message.vi"("Priority Message? (F)"=TRUE, "Message"="Pre-Exit", "Message Queue"=w556) -> ("error out"=w555:errorcluster, "dup Message Queue"=w554:refnum<queue>)  [unwired: 7 in]
      }
      event User Event {
        # "The Message Handling Loop processed an \"Exit\" message, which fired this event to stop the Event Handling Loop."
        n185 = event-data() -> ()  [unwired: 1 in, 1 out]
        n186 = local write "Messages"("\"Exit\" button pressed" ("VI Stopped")) -> ()
      }
    }
    n187 = call "Error Handler - Event Handling Loop.vi"("error in (no error)"=w502, "Message Queue"=w500) -> ("dup error in"=w499:errorcluster)  [unwired: 8 in, 1 out]
  }
  n188 = Unregister For Events(event registration refnum=w20, error in=w4) -> (error out=w21:errorcluster)
  n189 = Merge Errors(w21, w24, w13) -> (w22:errorcluster)
  n190 = call "Destroy User Event - Stop.vi"("error in (no error)"=w22, "User Event - Stop"=w17) -> ()  [unwired: 9 in, 1 out]
